vi "testCheckData.vi"(8 "error in (no error)":errorcluster) -> (0 "error out":errorcluster)   [LabVIEW 2018]
uses:
  src/CmpTool/checkData_priority.vi
  src/CmpTool/checkData_summaryState.vi
  <vilib>/addons/_JKI Toolkits/Caraya/classes/Assert/Assert True.vi
  <vilib>/addons/_JKI Toolkits/Caraya/classes/Assert/Assert False.vi
  <vilib>/addons/_JKI Toolkits/Caraya/classes/Test/Test.lvclass
  <vilib>/addons/_JKI Toolkits/Caraya/classes/Assert/Assert.lvclass
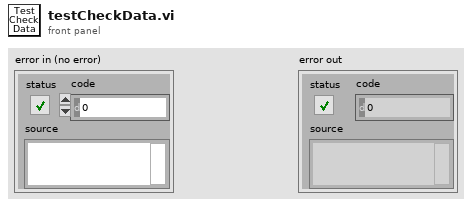
[diagram p1: front panel]
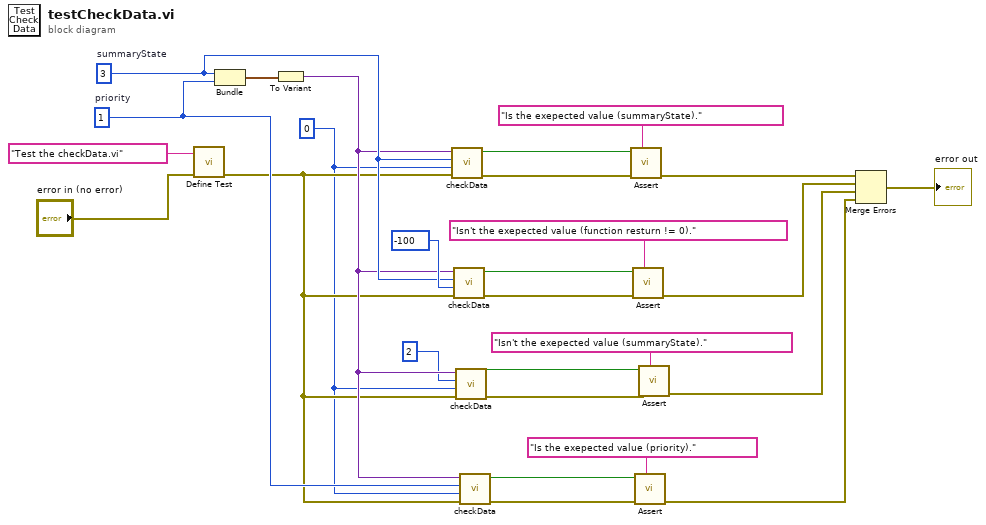
[diagram p0: block diagram]
diagram:
  w6 = 0
  w22 = 1  # priority
  w23 = 3  # summaryState
  n1 = call <vilib>:"Define Test.vi"("error in (no error)"="error in (no error)", "Label (VI Title)"="Test the checkData.vi") -> ("error out"=w7:errorcluster)  [unwired: 9 in]
  n2 = Bundle("summaryState"=w23, "priority"=w22) -> (w25:cluster{"summaryState":i32, "priority":i32})  [unwired: 1 in]
  n3 = To Variant(anything=w25) -> (Variant=w8:variant)
  n4 = call-poly "checkData.vi"("error in (no error)"=w7, "function return"=w6, "valExpect"=w23, "variant"=w8) -> ("error out"=w21:errorcluster, "isExpected"=w20:bool)  [unwired: 6 in]
  n5 = call-poly "checkData.vi"("error in (no error)"=w7, "function return"=-100, "valExpect"=w23, "variant"=w8) -> ("error out"=w19:errorcluster, "isExpected"=w18:bool)  [unwired: 6 in]
  n6 = call-poly "checkData.vi"("error in (no error)"=w7, "function return"=w6, "valExpect"=2, "variant"=w8) -> ("error out"=w4:errorcluster, "isExpected"=w3:bool)  [unwired: 6 in]
  n7 = call-poly "checkData.vi"("error in (no error)"=w7, "function return"=w6, "valExpect"=w22, "variant"=w8) -> ("error out"=w17:errorcluster, "isExpected"=w16:bool)  [unwired: 6 in]
  n8 = call-poly <vilib>:"Assert.vi"("Label"="Is the exepected value (summaryState).", "error in (no error)"=w21, "True?"=w20) -> ("error out"=w15:errorcluster)  [unwired: 8 in]
  n9 = call-poly <vilib>:"Assert.vi"("Label"="Isn't the exepected value (function resturn != 0).", "error in (no error)"=w19, "False?"=w18) -> ("error out"=w14:errorcluster)  [unwired: 8 in]
  n10 = call-poly <vilib>:"Assert.vi"("Label"="Is the exepected value (priority).", "error in (no error)"=w17, "True?"=w16) -> ("error out"=w9:errorcluster)  [unwired: 8 in]
  n11 = call-poly <vilib>:"Assert.vi"("Label"="Isn't the exepected value (summaryState).", "error in (no error)"=w4, "False?"=w3) -> ("error out"=w2:errorcluster)  [unwired: 8 in]
  n12 = Merge Errors(w15, w14, w2, w9) -> (→"error out":errorcluster)
